vi "CaracterizacionOrg.vi"() -> ()   [LabVIEW 2015]
uses:
  EnumEstados1.ctl
  <vilib>/Analysis/3filter.llb/Filter Passband Type.ctl
  <vilib>/Analysis/baseanly.llb/IIR Cascade Filter (DBL).vi
  <vilib>/Analysis/NI_AALBase.lvlib
  <vilib>/Utility/NIReport.llb/NI_report.lvclass
  <vilib>/addons/_office/NI_ReportGenerationToolkit.lvlib
  <vilib>/addons/_office/excel.llb/Excel Easy Table (str).vi
panel:
  in  "Numeric Control":dbl=0.01 format="%.2f"
  in  "order":i32=2
  in  "Stop Button":bool
  in  "Blank Button 2":bool
  in  "Blank Button":bool
  out "Eficiencia:":dbl
  out "Factor de Llenado:":dbl
  in  "Ok":bool
  in  "Save Button":bool
  in  "Guardar en:":path
  in  "Dispositivo:":enum16{"OLED", "OFET", "OPV"}(ring)
  in  "Voltaje final:":dbl
  in  "Voltaje inicial:":dbl
  out "Voltage-Current Characterization:":cluster{dbl[], "Filtered X":dbl[]}(graph)
  in  "Paso":dbl
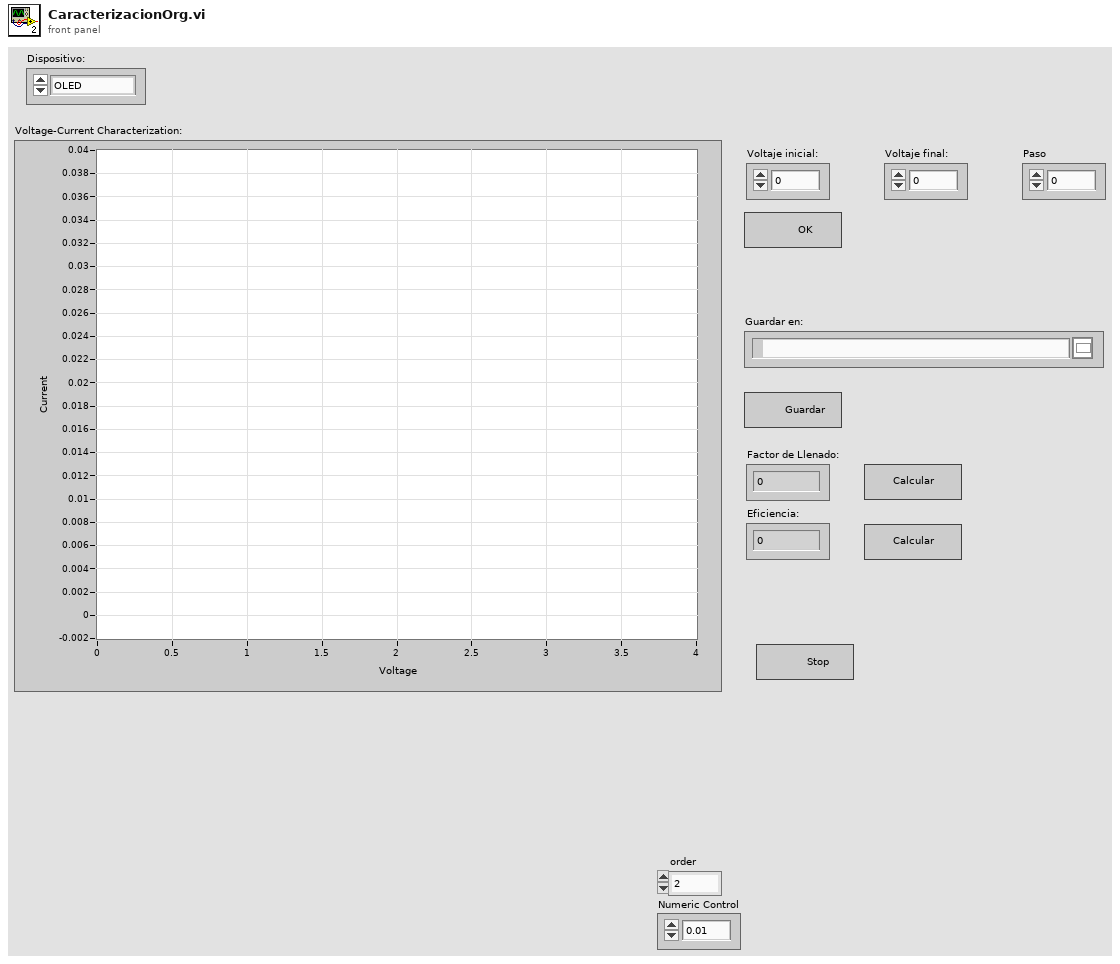
[diagram p1: front panel]
types:
  T1 = typedef "EnumEstados1.ctl" = enum16{"Inicio", "LecturaDatos", "Cierre"}
  T2 = typedef "NI_AALBase.lvlib/Filter Passband Type.ctl" = enum32{"Lowpass", "Highpass", "Bandpass", "Bandstop"}
  T3 = enum16{"Standard Report", "HTML", "Word", "Excel"}
  T4 = enum16{"maximized", "minimized", "normal", "no change"}
  T5 = enum16{"open", "open or create", "create or replace", "create", "open (read-only)"}
  T6 = cluster{"task out":refnum<k21>, "error out":errorcluster}
  T7 = cluster{"filter structure":enum32{"IIR 2nd Order", "IIR 4th Order"}, "Reverse Coefficients":dbl[], "Forward Coefficients":dbl[]}
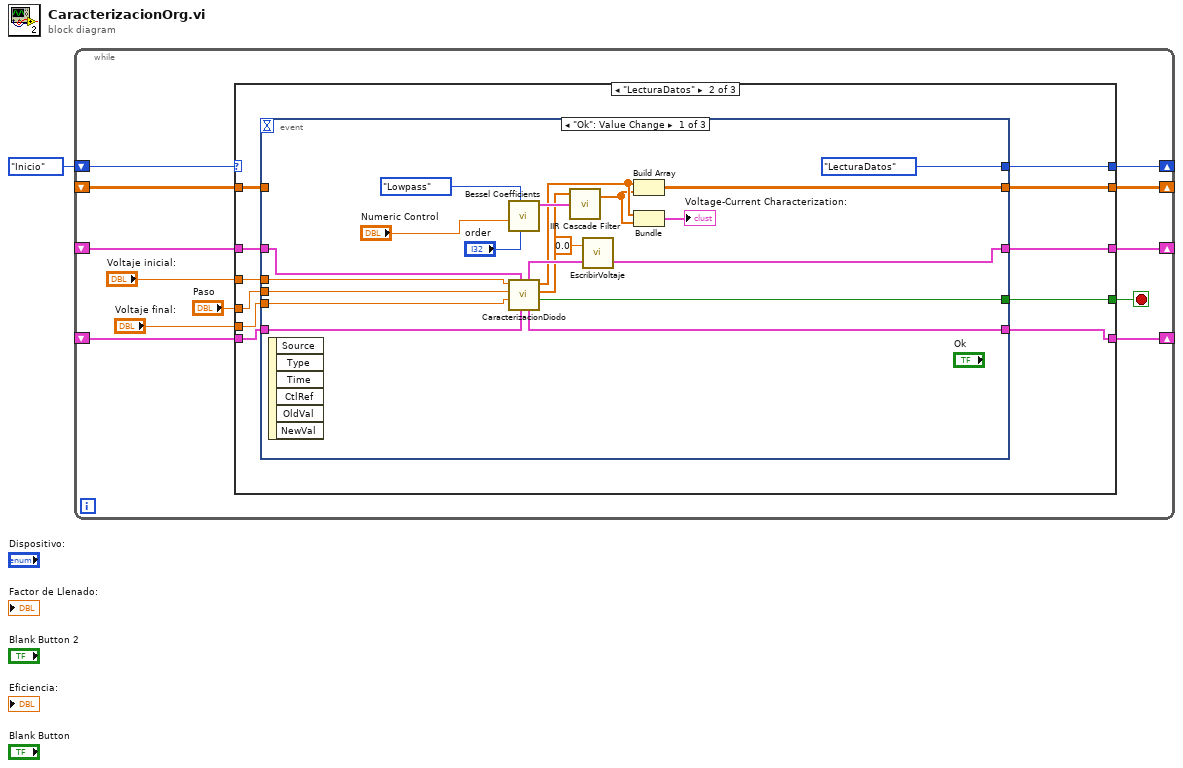
[diagram p0: block diagram]
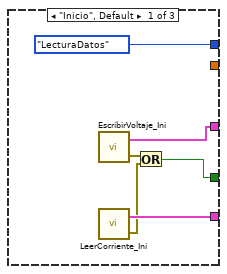
[diagram p2: hidden frame]
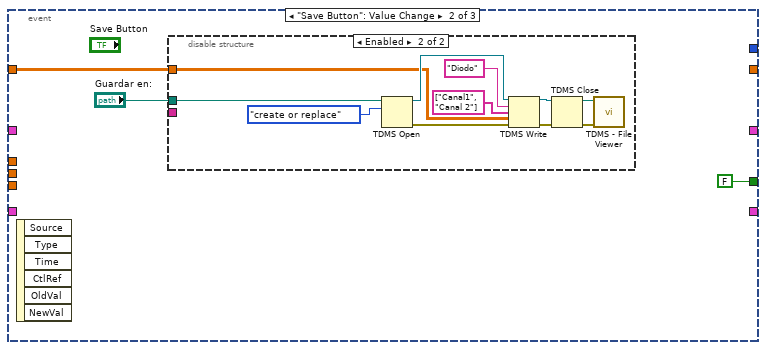
[diagram p3: hidden frame]
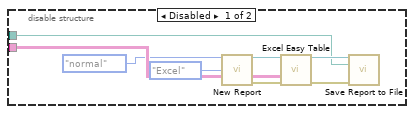
[diagram p4: hidden frame]
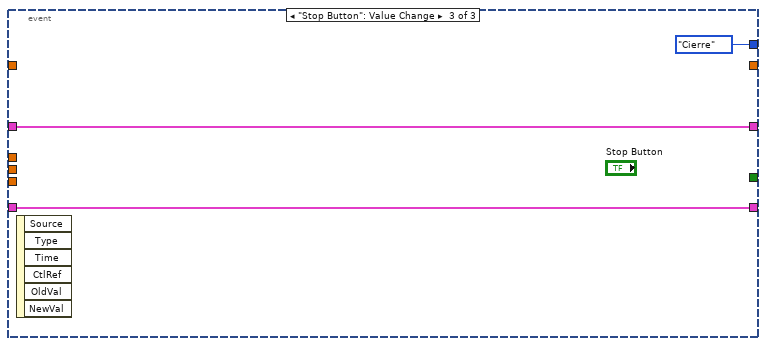
[diagram p5: hidden frame]
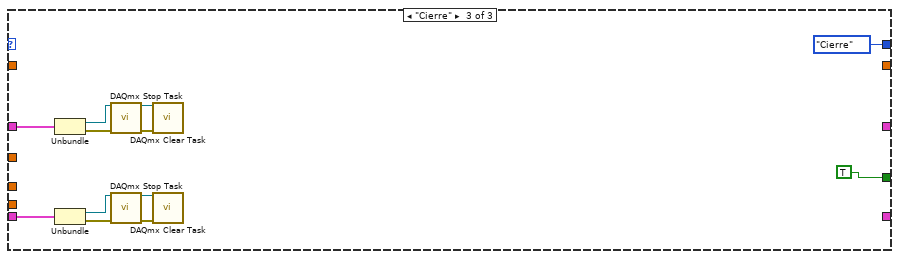
[diagram p6: hidden frame]
diagram:
  n1 = while {
    shift-right: [w5] -> _
    shift-left: EnumEstados1."Inicio" -> [w13]
    shift-right: [w9] -> _
    shift-left: _ -> [w8]
    shift-right: [w7] -> _
    shift-left: _ -> [w6]
    shift-right: [w4] -> _
    shift-left: _ -> [w3]
    stop <- w2 stop-if-true
    n2 = case shown="\"LecturaDatos\"" w13 {
      tunnel: "Voltaje final:" -> [_ w30 _]
      tunnel: "Voltaje inicial:" -> [_ w24 _]
      tunnel: "Paso" -> [_ w25 _]
      tunnel: [w18 w28 _] -> w9
      tunnel: w8 -> [_ w29 w83]
      tunnel: [w17 w26 _] -> w7
      tunnel: w6 -> [_ w27 w82]
      tunnel: [EnumEstados1."LecturaDatos" w23 EnumEstados1."Cierre"] -> w5
      tunnel: [_ w22 _] -> w4
      tunnel: w3 -> [_ w21 _]
      tunnel: [w14 w20 TRUE] -> w2
      frame "Inicio", Default {
        n3 = call "EscribirVoltaje_Ini.vi"() -> ("error out"=w16:errorcluster, "cluster"=w18:T6)  [unwired: 2 in]
        n4 = call "LeerCorriente_Ini.vi"() -> ("error out"=w15:errorcluster, "output cluster"=w17:T6)  [unwired: 2 in]
        n5 = Or(x=w16, y=w15) -> (x .or. y?=w14:bool)
      }
      frame "LecturaDatos" {
        n6 = event shown="[0] \"Ok\": Value Change" {
          selector: _ -> [_ _ _]
          dyn-events: _ -> [_ _ _]
          timeout: _ -> [_ _ _]
          tunnel: w30 -> [w41 _ _]
          tunnel: w29 -> [w40 _ w75]
          tunnel: [w46 _ w75] -> w28
          tunnel: w27 -> [w39 _ w74]
          tunnel: [w36 _ w74] -> w26
          tunnel: w25 -> [w42 _ _]
          tunnel: w24 -> [w43 _ _]
          tunnel: [EnumEstados1."LecturaDatos" _ EnumEstados1."Cierre"] -> w23
          tunnel: [w33 _ _] -> w22
          tunnel: w21 -> [_ w52 _]
          tunnel: [w31 FALSE _] -> w20
          event "Ok": Value Change {
            n7 = event-data() -> ()  [unwired: 1 in, 6 out]
            n8 = call <vilib>:"Bessel Coefficients.vi"("order"="order", "filter type"=Filter_Passband_Type."Lowpass", "low cutoff freq: fl"="Numeric Control") -> ("IIR Filter Cluster"=w49:T7)  [unwired: 7 in, 1 out]
            n9 = call "CaracterizacionDiodo.vi"("Corriente"=w39, "Voltaje"=w40, "Voltaje final:"=w41, "Paso"=w42, "Voltaje inicial:"=w43) -> ("Error?"=w31:bool, 2:"Corriente"=w34:dbl[], 3:"Voltaje"=w37:dbl[], 4:"Corriente"=w36:T6, 5:"Voltaje"=w38:T6)  [unwired: 2 in]
            n10 = call-poly <vilib>:"IIR Cascade Filter.vi"("IIR Filter Cluster"=w49, "X"=w34) -> ("Filtered X"=w32:dbl[])  [unwired: 1 in, 1 out]
            n11 = call "EscribirVoltaje.vi"("cluster"=w38, "data"=0.0) -> ("Cluster"=w46:T6)  [unwired: 1 out]
            n12 = Build Array(w37, w32) -> (w33:dbl[][])
            n13 = Bundle("Voltaje"=w37, "Filtered X"=w32) -> (→"Voltage-Current Characterization:":cluster{"Voltaje":dbl[], "Filtered X":dbl[]})  [unwired: 1 in]
          }
          event "Save Button": Value Change {
            n14 = event-data() -> ()  [unwired: 1 in, 6 out]
            n15 = disable-structure shown="Enabled" {
              disable-tunnel: _ -> [w59 _]
              disable-tunnel: "Guardar en:" -> [w54 w65]
              disable-tunnel: w52 -> [_ w62]
              frame Disabled {
                n16 = call <vilib>:"New Report.vi"("window state (normal)"=T4."normal", "report type"=T3."Excel") -> ("report out"=w61:refnum<class "NI_report.lvclass">, "error out"=w60:errorcluster)  [unwired: 12 in]
                n17 = call-poly <vilib>:"Excel Easy Table.vi"("report in"=w61, "text data"=w59, "error in (no error)"=w60) -> ("report out"=w58:refnum<class "NI_report.lvclass">, "error out"=w57:errorcluster)  [unwired: 8 in, 3 out]
                n18 = call-dynamic "Save Report to File.vi"("report in"=w58, "report file path"=w54, "error in (no error)"=w57) -> ()  [unwired: 11 in, 2 out]
              }
              frame Enabled {
                n19 = TDMS Open(10:T5."create or replace" ("operation (0:open)"), 11:w65) -> (0:w69:errorcluster, 3:w66:refnum<k34>)  [unwired: 5 in]
                n20 = TDMS Write(0:w66, 5:"Diodo" ("group name in (Untitled)"), 7:string[] ["Canal1", "Canal 2"] ("channel name(s) in (Untitled)"), 9:w62, 11:w69) -> (4:w67:refnum<k34>, 15:w68:errorcluster)  [unwired: 1 in, 2 out]
                n21 = TDMS Close(8:w68, 11:w67) -> (0:w64:errorcluster, 3:w63:path)
                n22 = call <vilib>:"TDMS - File Viewer.vi"("error in (no error)"=w64, "file path"=w63) -> ()  [unwired: 4 in, 2 out]
              }
            }
          }
          event "Stop Button": Value Change {
            n23 = event-data() -> ()  [unwired: 1 in, 6 out]
          }
        }
      }
      frame "Cierre" {
        n24 = Unbundle(w83) -> ("task out"=w81:refnum<k21>, "error out"=w80:errorcluster)
        n25 = Unbundle(w82) -> ("task out"=w79:refnum<k21>, "error out"=w78:errorcluster)
        n26 = call <vilib>:"DAQmx Stop Task.vi"("task/channels in"=w81, "error in"=w80) -> ("task out"=w87:refnum<k21>, "error out"=w86:errorcluster)  [unwired: 12 in]
        n27 = call <vilib>:"DAQmx Stop Task.vi"("task/channels in"=w79, "error in"=w78) -> ("task out"=w85:refnum<k21>, "error out"=w84:errorcluster)  [unwired: 12 in]
        n28 = call <vilib>:"DAQmx Clear Task.vi"("task in"=w87, "error in"=w86) -> ()  [unwired: 13 in, 1 out]
        n29 = call <vilib>:"DAQmx Clear Task.vi"("task in"=w85, "error in"=w84) -> ()  [unwired: 13 in, 1 out]
      }
    }
  }
